vi "Check Hardware Serial Number.vi"(11 "Error In":errorcluster) -> (4 "Hardware Serial Number Changed?":bool, 6 "Hardware Calibration Date Exceeded?":bool, 8 "Changed Instrument List":string, 15 "Error Out":errorcluster)   [LabVIEW 2010]
uses:
  <vilib>/Utility/miscctls.llb/LVDateTimeRec.ctl
  <vilib>/Utility/file.llb/Read From Spreadsheet File (string).vi
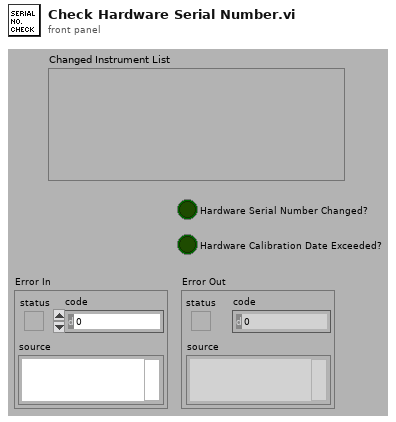
[diagram p1: front panel]
types:
  T1 = typedef "LVDateTimeRec.ctl" = cluster{"fractional second":dbl, "second":i32, "minute":i32, "hour":i32, "day of month":i32, "month":i32, "year":i32, "day of week":i32, "day of year":i32, "DST":i32}
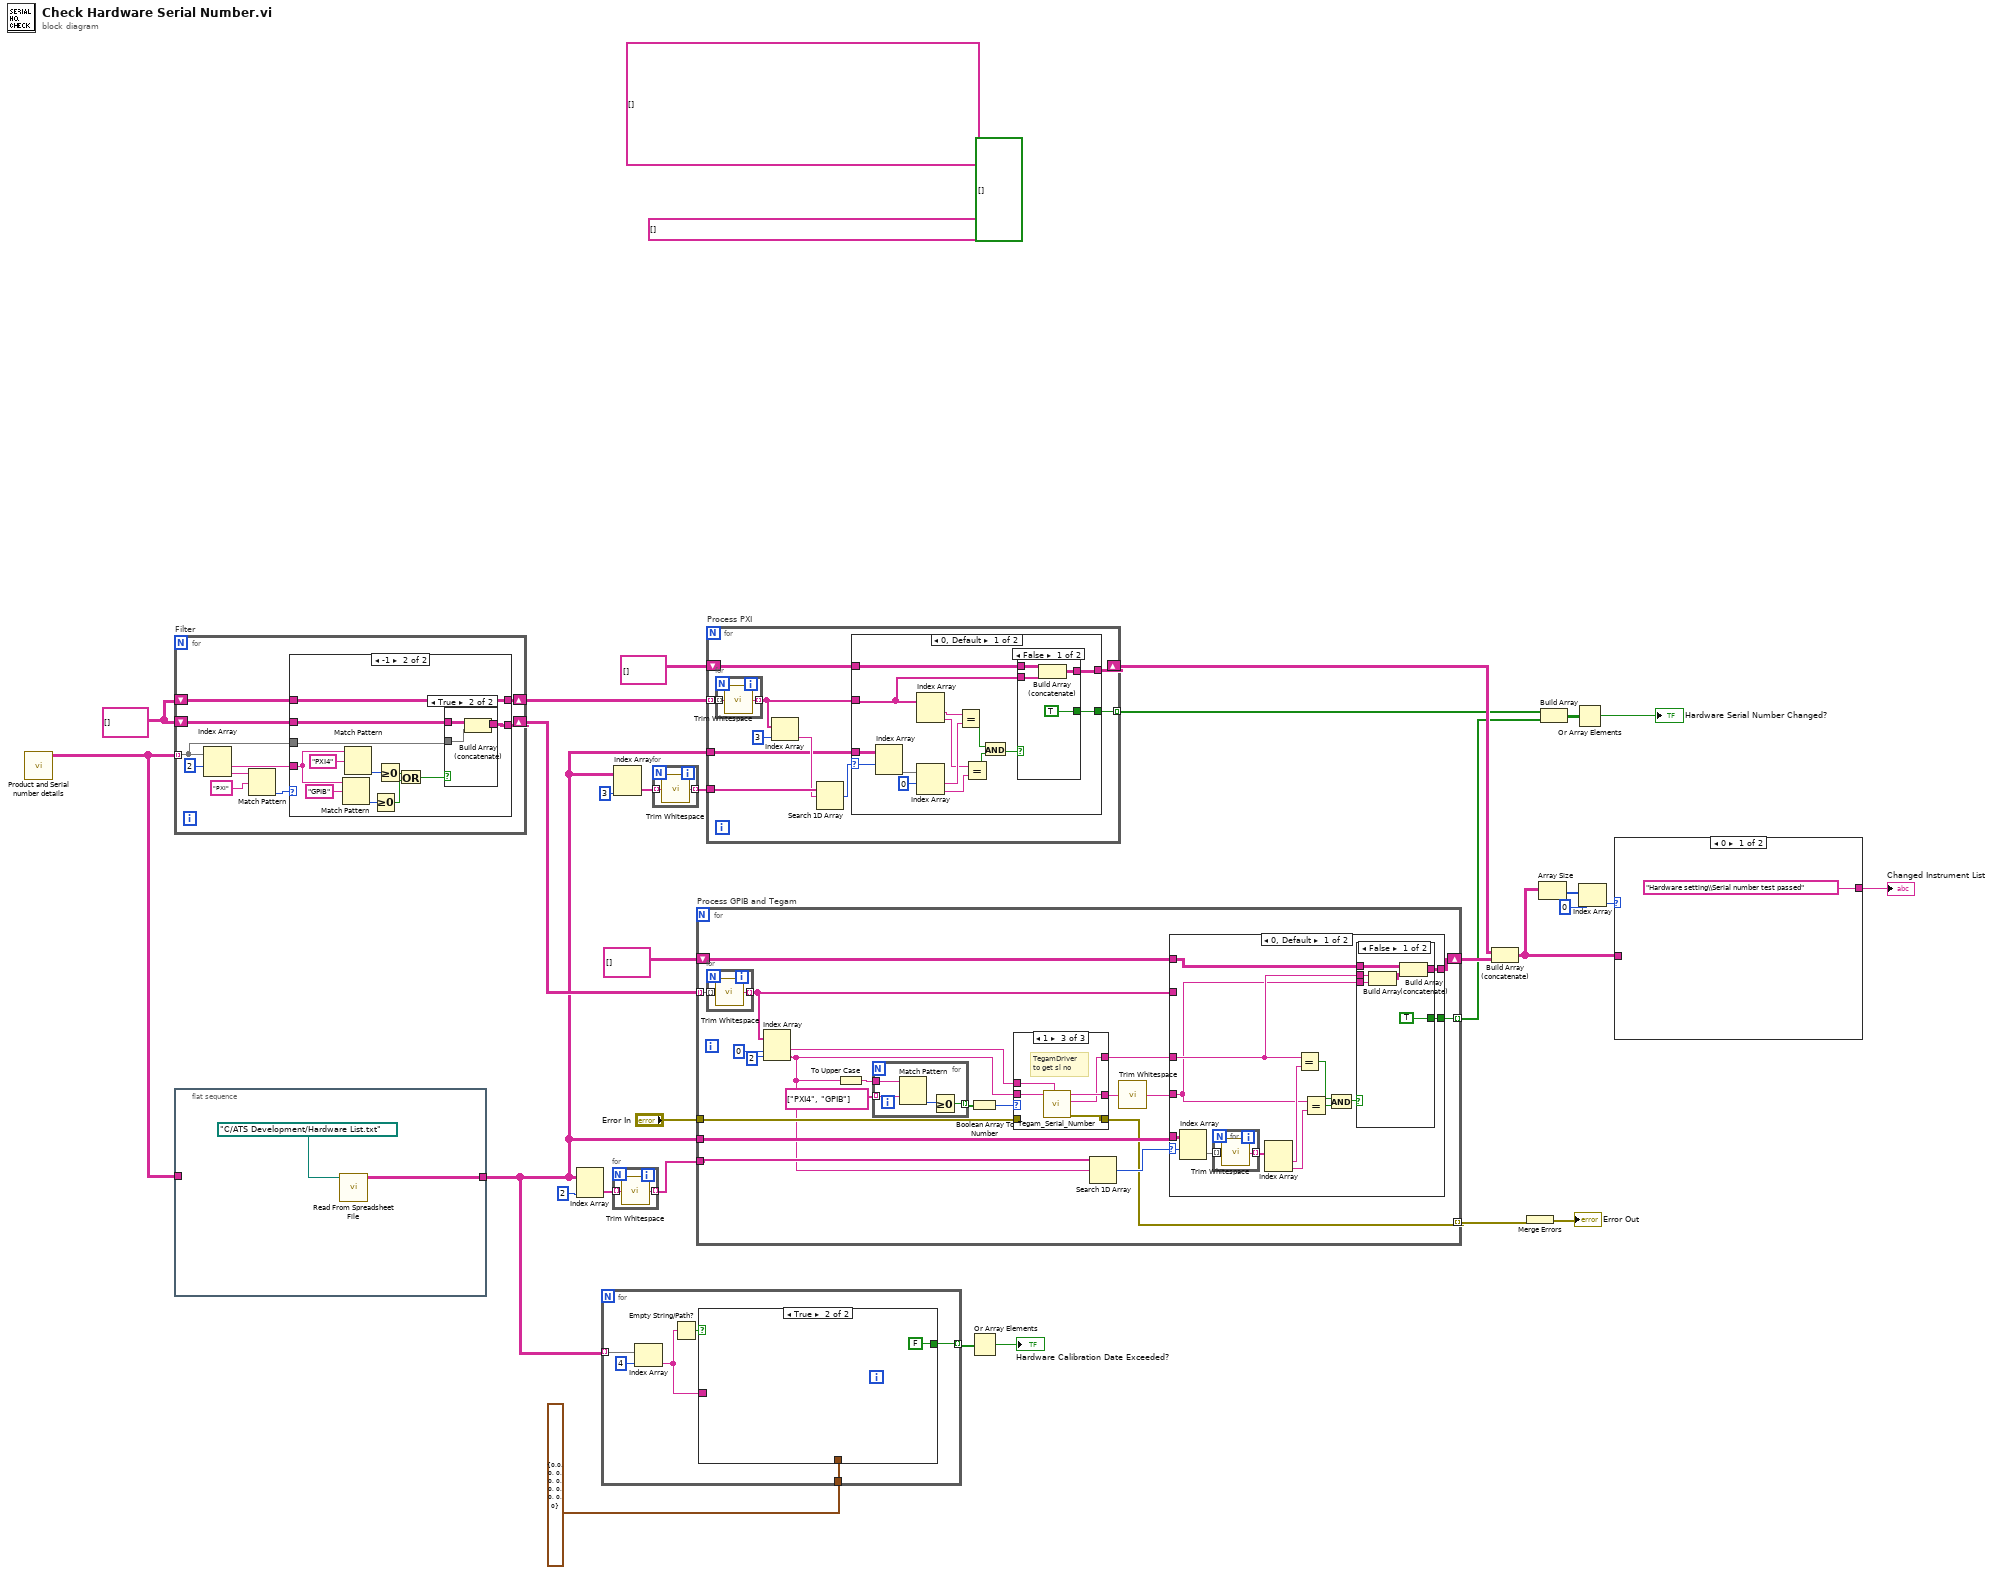
[diagram p0: block diagram]
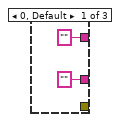
[diagram p2: hidden frame]
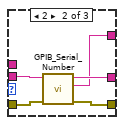
[diagram p3: hidden frame]
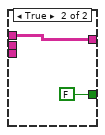
[diagram p4: hidden frame]
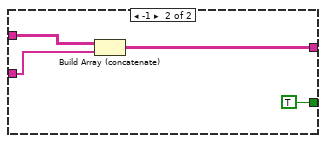
[diagram p5: hidden frame]
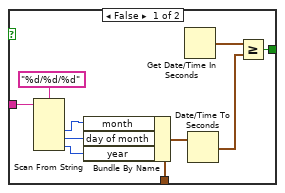
[diagram p6: hidden frame]
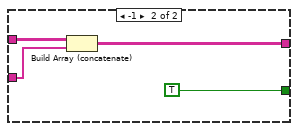
[diagram p8: hidden frame]
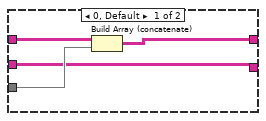
[diagram p9: hidden frame]
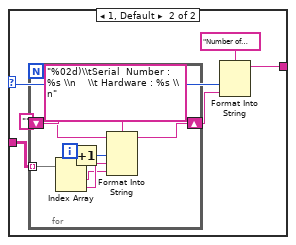
[diagram p11: hidden frame]
diagram:
  w26 = string[][] [] ("Lookup Table")
  (unwired) string[] []
  (unwired) string[][] []
  (unwired) bool[] []
  n1 = call "Product and Serial number details.vi"() -> ("Product and Serial Number"=w6:string[][])  [unwired: 10 in, 1 out]
  n2 = for "Filter" {
    tunnel: w6 -> [w34] mode=indexing
    shift-right: [w33] -> w22
    shift-left: w26 -> [w35]
    shift-right: [w31] -> w25
    shift-left: w26 -> [w32]
    n3 = Index Array(array=w34, index #1=2 ("index")) -> (element #1=w36:string, element #2=w39:string)  [unwired: 1 in]
    n4 = Match Pattern(string=w39, regular expression="PXI") -> (offset past match=w37:i32)  [unwired: 1 in, 3 out]
    n5 = case shown="-1" w37 {
      tunnel: w36 -> [_ w54]
      tunnel: w35 -> [w41 w48]
      tunnel: w34 -> [w44 w47]
      tunnel: [w41 w46] -> w33
      tunnel: w32 -> [w43 w45]
      tunnel: [w42 w45] -> w31
      frame 0, Default {
        n6 = Build Array (concatenate)(w43, w44) -> (w42:string[][])
      }
      frame -1 {
        n7 = Match Pattern(string=w54, regular expression="GPIB") -> (offset past match=w52:i32)  [unwired: 1 in, 3 out]
        n8 = Match Pattern(string=w54, regular expression="PXI4") -> (offset past match=w53:i32)  [unwired: 1 in, 3 out]
        n9 = Greater Or Equal To 0?(x=w52) -> (x >= 0?=w51:bool)
        n10 = Greater Or Equal To 0?(x=w53) -> (x >= 0?=w50:bool)
        n11 = Or(x=w50, y=w51) -> (x .or. y?=w49:bool)
        n12 = case shown="True" w49 {
          tunnel: w48 -> [w57 w60]
          tunnel: w47 -> [_ w59]
          tunnel: [w57 w58] -> w46
          frame False {
          }
          frame True {
            n13 = Build Array (concatenate)(w60, w59) -> (w58:string[][])
          }
        }
      }
    }
  }
  n14 = flat-sequence {
    tunnel: [w61] -> w3
    tunnel: w6 -> [_]
    frame #0 {
      n15 = call-poly <vilib>:"Read From Spreadsheet File.vi"("file path (dialog if empty)"=path "C:/ATS Development/Hardware List.txt") -> ("all rows"=w61:string[][])  [unwired: 6 in, 4 out]
    }
  }
  n16 = Index Array(array=w3, index (col)=2 ("disabled index (col)")) -> (element=w8:string[])  [unwired: 1 in]
  n17 = for {
    tunnel: T1 {"fractional second"=0.0, "second"=0, "minute"=0, "hour"=0, "day of month"=0, "month"=0, "year"=0, "day of week"=0, "day of year"=0, "DST"=0} ("date time rec") -> [w67]
    tunnel: w3 -> [w64] mode=indexing
    tunnel: [w63] -> w4 mode=indexing
    n18 = Index Array(array=w64, index=4) -> (element=w65:string)
    n19 = Empty String/Path?(string/path=w65) -> (empty?=w66:bool)
    n20 = case shown="True" w66 {
      tunnel: w67 -> [w77 _]
      tunnel: w65 -> [w72 _]
      tunnel: [w69 FALSE] -> w63
      frame False {
        n21 = Scan From String(format string="%d/%d/%d", input string=w72) -> (output 1=w75:i32, output 2=w74:i32, output 3=w73:i32)  [unwired: 5 in, 3 out]
        n22 = Bundle By Name(cluster=w77, "month"=w75, "day of month"=w74, "year"=w73) -> (w76:T1)
        n23 = Get Date/Time In Seconds() -> (seconds since 1Jan1904=w71:timestamp)
        n24 = Date/Time To Seconds(2:w76) -> (0:w70:timestamp)  [unwired: 1 in]
        n25 = Greater Or Equal?(x=w71, y=w70) -> (x >= y?=w69:bool)
      }
      frame True {
      }
    }
  }
  n26 = for {
    tunnel: w8 -> [w81] mode=indexing
    tunnel: [w80] -> w7 mode=indexing
    n27 = call <vilib>:"Trim Whitespace.vi"("string"=w81) -> ("trimmed string"=w80:string)  [unwired: 1 in]
  }
  n28 = Index Array(array=w3, index (col)=3 ("disabled index (col)")) -> (element=w10:string[])  [unwired: 1 in]
  n29 = for {
    tunnel: w10 -> [w83] mode=indexing
    tunnel: [w82] -> w9 mode=indexing
    n30 = call <vilib>:"Trim Whitespace.vi"("string"=w83) -> ("trimmed string"=w82:string)  [unwired: 1 in]
  }
  n31 = for "Process GPIB and Tegam" {
    tunnel: w22 -> [w89] mode=indexing
    tunnel: w3 -> [w101]
    tunnel: w7 -> [w93]
    shift-right: [w102] -> w15
    shift-left: string[][] [] ("Lookup Table") -> [w103]
    tunnel: "Error In" -> [w96]
    tunnel: [w92] -> w18 mode=indexing
    tunnel: [w91] -> w13 mode=indexing
    n32 = for {
      tunnel: w89 -> [w106] mode=indexing
      tunnel: [w105] -> w88 mode=indexing
      n33 = call <vilib>:"Trim Whitespace.vi"("string"=w106) -> ("trimmed string"=w105:string)  [unwired: 1 in]
    }
    n34 = Index Array(array=w88, index #1=0 ("index"), index #2=2 ("index")) -> (element #1=w84:string, element #2=w85:string)
    n35 = To Upper Case(1:w85) -> (0:w100:string)
    n36 = for {
      tunnel: w100 -> [w122]
      tunnel: string[] ["PXI4", "GPIB"] -> [w121] mode=indexing
      tunnel: [w119] -> w98 mode=indexing
      n37 = Match Pattern(string=w122, regular expression=w121) -> (offset past match=w120:i32)  [unwired: 1 in, 3 out]
      n38 = Greater Or Equal To 0?(x=w120) -> (x >= 0?=w119:bool)
    }
    n39 = Boolean Array To Number(Boolean array=w98) -> (number=w97:u32)
    n40 = case shown="1" w97 {
      tunnel: ["" ("Serial Number") w110 w117] -> w95
      tunnel: w85 -> [_ w112 w115]
      tunnel: [_ w113 w118] -> w92
      tunnel: w96 -> [_ w111 _]
      tunnel: ["" ("Model") w109 w116] -> w90
      tunnel: w84 -> [_ _ w114]
      frame 0, Default {
      }
      frame 2 {
        n41 = call "GPIB_Serial_Number.vi"("Error In"=w111, "GPIB Address"=w112) -> ("Error Out"=w113:errorcluster, "Model"=w109:string, "Serial Number"=w110:string)  [unwired: 7 in]
      }
      frame 1 {
        # "TegamDriver\nto get sl no"
        n42 = call "Tegam_Serial_Number.vi"("Expected Model"=w114, "GPIB Address"=w115) -> ("Error Out"=w118:errorcluster, "Model"=w116:string, "Serial Number"=w117:string)  [unwired: 7 in]
      }
    }
    n43 = Search 1D Array(1D array=w93, element=w85) -> (index of element=w104:i32)  [unwired: 1 in]
    n44 = call <vilib>:"Trim Whitespace.vi"("string"=w95) -> ("trimmed string"=w94:string)  [unwired: 1 in]
    n45 = case shown="0, Default" w104 {
      selector: w104 -> [w135 _]
      tunnel: w88 -> [_ w150]
      tunnel: w103 -> [w129 w149]
      tunnel: [w128 w148] -> w102
      tunnel: w101 -> [w136 _]
      tunnel: w94 -> [w125 _]
      tunnel: [w127 TRUE] -> w91
      tunnel: w90 -> [w126 _]
      frame 0, Default {
        n46 = Index Array(array=w136, index (row)=w135) -> (element=w124:string[])  [unwired: 1 in]
        n47 = for {
          tunnel: w124 -> [w138] mode=indexing
          tunnel: [w137] -> w123 mode=indexing
          n48 = call <vilib>:"Trim Whitespace.vi"("string"=w138) -> ("trimmed string"=w137:string)  [unwired: 1 in]
        }
        n49 = Index Array(array=w123) -> (element #1=w134:string, element #2=w133:string)  [unwired: 2 in]
        n50 = Equal?(x=w126, y=w134) -> (x = y?=w132:bool)
        n51 = Equal?(x=w125, y=w133) -> (x = y?=w131:bool)
        n52 = And(x=w132, y=w131) -> (x .and. y?=w130:bool)
        n53 = case shown="False" w130 {
          tunnel: w129 -> [w144 w146]
          tunnel: [w143 w146] -> w128
          tunnel: [TRUE FALSE] -> w127
          tunnel: w126 -> [w141 _]
          tunnel: w125 -> [w139 _]
          frame False {
            n54 = Build Array(w141, w139) -> (w140:string[])
            n55 = Build Array (concatenate)(w144, w140) -> (w143:string[][])
          }
          frame True {
          }
        }
      }
      frame -1 {
        n56 = Build Array (concatenate)(w149, w150) -> (w148:string[][])
      }
    }
  }
  n57 = for "Process PXI" {
    tunnel: w25 -> [w152] mode=indexing
    tunnel: w3 -> [w154]
    tunnel: w9 -> [w160]
    shift-right: [w155] -> w17
    shift-left: string[][] [] ("Lookup Table") -> [w156]
    tunnel: [w153] -> w16 mode=indexing
    n58 = for {
      tunnel: w152 -> [w162] mode=indexing
      tunnel: [w161] -> w151 mode=indexing
      n59 = call <vilib>:"Trim Whitespace.vi"("string"=w162) -> ("trimmed string"=w161:string)  [unwired: 1 in]
    }
    n60 = Index Array(array=w151, index=3) -> (element=w159:string)
    n61 = Search 1D Array(1D array=w160, element=w159) -> (index of element=w158:i32)  [unwired: 1 in]
    n62 = case shown="0, Default" w158 {
      selector: w158 -> [w176 _]
      tunnel: w151 -> [w165 w186]
      tunnel: w156 -> [w166 w185]
      tunnel: [w164 w184] -> w155
      tunnel: w154 -> [w177 _]
      tunnel: [w163 TRUE] -> w153
      frame 0, Default {
        n63 = Index Array(array=w177, index (row)=w176) -> (element=w175:string[])  [unwired: 1 in]
        n64 = Index Array(array=w165) -> (element #1=w173:string, element #2=w170:string)  [unwired: 2 in]
        n65 = Index Array(array=w175, index #1=0 ("index")) -> (element #1=w172:string, element #2=w171:string)  [unwired: 1 in]
        n66 = Equal?(x=w173, y=w172) -> (x = y?=w169:bool)
        n67 = Equal?(x=w170, y=w171) -> (x = y?=w168:bool)
        n68 = And(x=w169, y=w168) -> (x .and. y?=w167:bool)
        n69 = case shown="False" w167 {
          tunnel: w166 -> [w181 w182]
          tunnel: w165 -> [w180 _]
          tunnel: [w179 w182] -> w164
          tunnel: [TRUE _] -> w163
          frame False {
            n70 = Build Array (concatenate)(w181, w180) -> (w179:string[][])
          }
          frame True {
          }
        }
      }
      frame -1 {
        n71 = Build Array (concatenate)(w185, w186) -> (w184:string[][])
      }
    }
  }
  n72 = Or Array Elements(Boolean array=w4) -> (logical OR=→"Hardware Calibration Date Exceeded?":bool)
  n73 = Build Array (concatenate)(w17, w15) -> (w14:string[][])
  n74 = Merge Errors(w18) -> (→"Error Out":errorcluster)
  n75 = Array Size(array=w14) -> (size(s)=w30:i32[])
  n76 = Build Array(w16, w13) -> (w12:bool[][])
  n77 = Or Array Elements(Boolean array=w12) -> (logical OR=→"Hardware Serial Number Changed?":bool)
  n78 = Index Array(array=w30, index=0) -> (element=w28:i32)
  n79 = case shown="0" w28 {
    selector: w28 -> [_ w193]
    tunnel: w14 -> [_ w192]
    tunnel: ["Hardware setting\\Serial number test passed" w188] -> w2
    frame 0 {
    }
    frame 1, Default {
      n80 = for {
        tunnel: w192 -> [w198] mode=indexing
        shift-right: [w200] -> w190
        shift-left: "" ("element") -> [w201]
        i -> [w199]
        n81 = Index Array(array=w198) -> (element #1=w194:string, element #2=w195:string)  [unwired: 2 in]
        n82 = Increment(x=w199) -> (x+1=w197:i32)
        n83 = Format Into String(format string="%02d)\\tSerial  Number : %s \\n    \\t Hardware : %s \\n", initial string=w201, w197, w195, w194) -> (resulting string=w200:string)  [unwired: 1 in, 1 out]
      }
      n84 = Format Into String(format string="Number of Hardware modified : %d\\n%s", w193, w190) -> (resulting string=w188:string)  [unwired: 2 in, 1 out]
    }
  }
  "Changed Instrument List" <- w2
